vi "Matrix Offset String.vi"(0 "ProgramList in":string[](array[string]), 1 "Matrix string":string, 2 "x":dbl, 3 "y":dbl, 4 "z":dbl) -> (14 "ProgramListOut":string[](array[string]), 15 "Matrix New String":string)   [LabVIEW 2014]
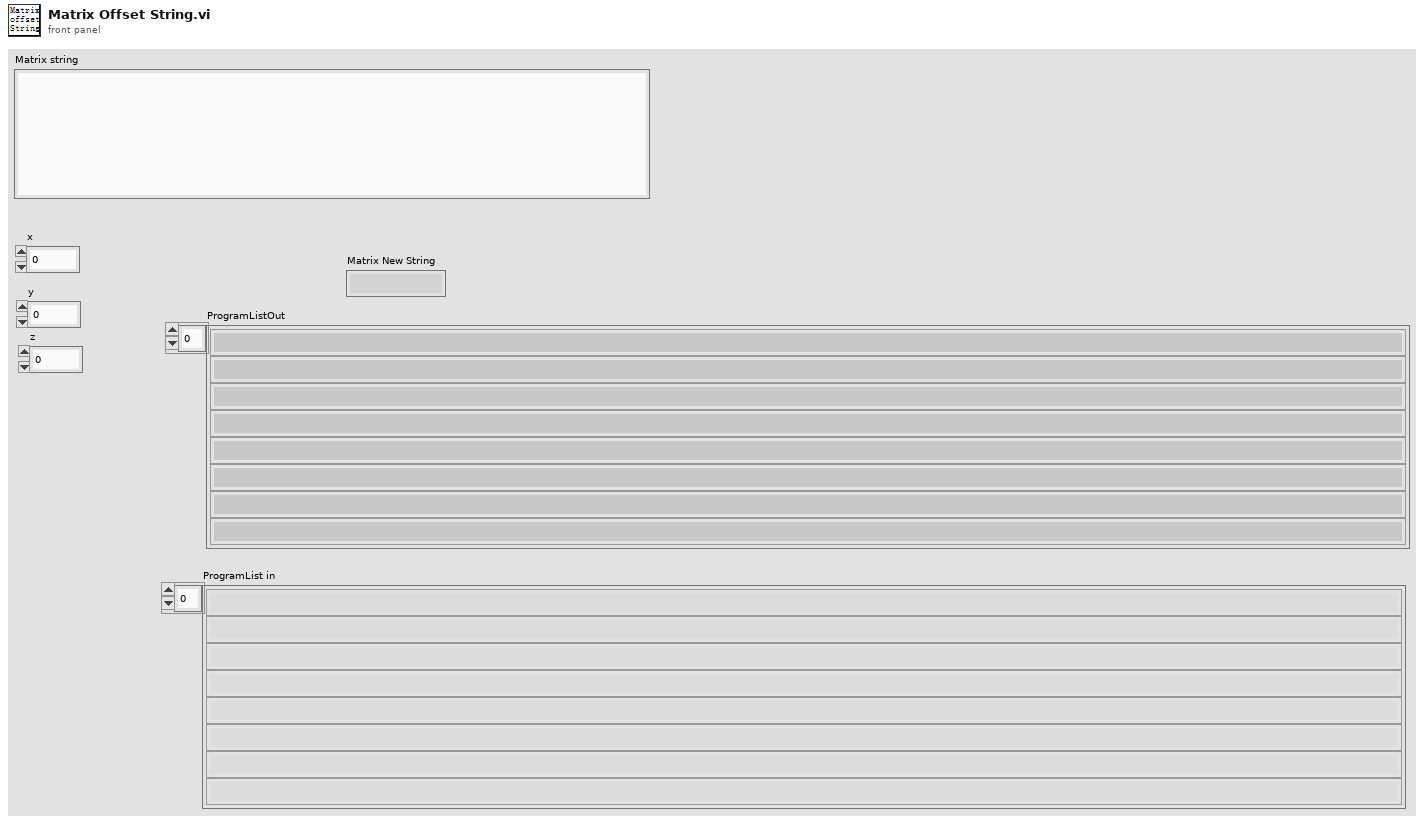
[diagram p1: front panel]
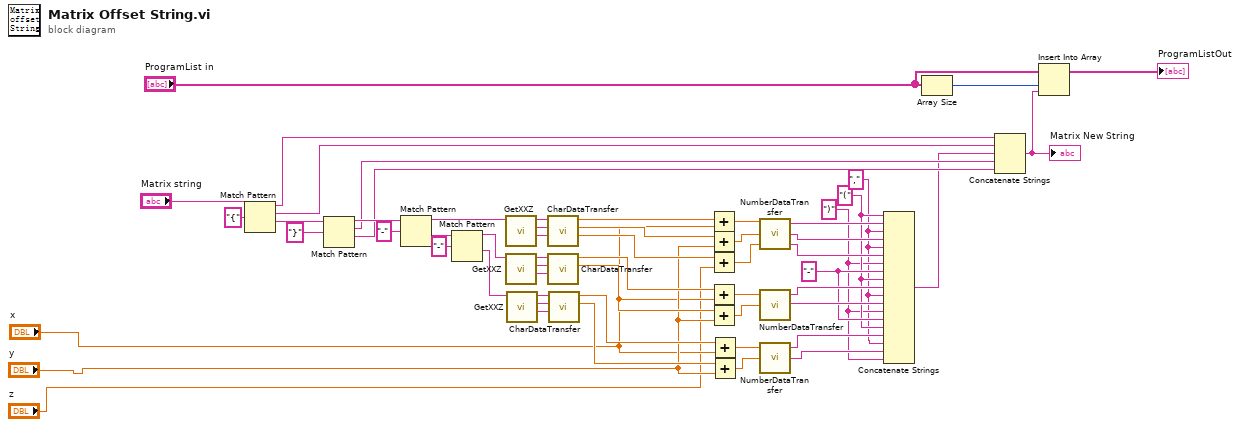
[diagram p0: block diagram]
diagram:
  w17 = "-" ("字符串")
  w13 = ")" ("字符串")
  w9 = "," ("字符串")
  w16 = "(" ("字符串")
  n1 = Match Pattern(string="Matrix string", regular expression="{" ("正则表达式")) -> (before substring=w24:string, match substring=w23:string, after substring=w55:string)  [unwired: 1 in, 1 out]
  n2 = Match Pattern(string=w55, regular expression="}" ("正则表达式")) -> (before substring=w39:string, match substring=w12:string, after substring=w11:string)  [unwired: 1 in, 1 out]
  n3 = Match Pattern(string=w39, regular expression="-" ("正则表达式")) -> (before substring=w48:string, after substring=w52:string)  [unwired: 1 in, 2 out]
  n4 = Match Pattern(string=w52, regular expression="-" ("正则表达式")) -> (before substring=w44:string, after substring=w40:string)  [unwired: 1 in, 2 out]
  n5 = call "GetXXZ.vi"("TrackIn"=w48) -> ("Z"=w50:string, "Y"=w51:string, "X"=w49:string)  [unwired: 6 in, 2 out]
  n6 = call "GetXXZ.vi"("TrackIn"=w44) -> ("Z"=w46:string, "Y"=w45:string, "X"=w47:string)  [unwired: 6 in, 2 out]
  n7 = call "GetXXZ.vi"("TrackIn"=w40) -> ("Z"=w42:string, "Y"=w43:string, "X"=w41:string)  [unwired: 6 in, 2 out]
  n8 = call "CharDataTransfer.vi"("Z"=w50, "Y"=w51, "X"=w49) -> ("Z"=w36:dbl, "Y"=w37:dbl, "X"=w38:dbl)  [unwired: 1 in, 1 out]
  n9 = call "CharDataTransfer.vi"("Z"=w46, "Y"=w45, "X"=w47) -> ("Y"=w34:dbl, "X"=w35:dbl)  [unwired: 1 in, 2 out]
  n10 = call "CharDataTransfer.vi"("Z"=w42, "Y"=w43, "X"=w41) -> ("Y"=w32:dbl, "X"=w33:dbl)  [unwired: 1 in, 2 out]
  n11 = Add(x=w38, y="x") -> (x+y=w31:dbl)
  n12 = Add(x=w37, y="y") -> (x+y=w30:dbl)
  n13 = Add(x=w36, y="z") -> (x+y=w29:dbl)
  n14 = Add(x=w35, y="x") -> (x+y=w28:dbl)
  n15 = Add(x=w34, y="y") -> (x+y=w27:dbl)
  n16 = Add(x=w33, y="x") -> (x+y=w26:dbl)
  n17 = Add(x=w32, y="y") -> (x+y=w25:dbl)
  n18 = call "NumberDataTransfer.vi"("Z"=w29, "Y"=w30, "X"=w31) -> ("Z"=w20:string, "Y"=w21:string, "X"=w22:string)
  n19 = call "NumberDataTransfer.vi"("Y"=w27, "X"=w28) -> ("Y"=w18:string, "X"=w19:string)  [unwired: 1 in, 1 out]
  n20 = call "NumberDataTransfer.vi"("Y"=w25, "X"=w26) -> ("Y"=w14:string, "X"=w15:string)  [unwired: 1 in, 1 out]
  n21 = Concatenate Strings(w16, w22, w9, w21, w9, w20, w13, w17, w16, w19, w9, w18, w13, w17, w16, w15, w9, w14, w13) -> (w10:string)
  n22 = Array Size(array="ProgramList in") -> (size(s)=w4:i32)
  n23 = Concatenate Strings(w24, w23, w10, w12, w11) -> (w1:string)
  "Matrix New String" <- w1
  n24 = Insert Into Array(array="ProgramList in", index=w4, new element=w1) -> (→"ProgramListOut":string[])
